vi "SequenceControl.vi"(0 "Sequence On? 2":bool, 5 "Counter 2":dbl, 7 "Sequence Instances 2":dbl, 9 "Sequence Storer":T1[][](array[typedef]) {"Amplitude Correction" step=0.1; "Line Trapping"."Phase Gradient" step=0.05; "Line Trapping"."Vector"."x" step=1e-06 format="%#_6p"; "Line Trapping"."Vector"."y" step=1e-06 format="%#_6p"; "Line Trapping"."Vector"."z" step=1e-06 format="%#_6p"; "NA Position"."r" step=1e-06; "NA Position"."y" step=1e-06; "NA Position"."x" step=1e-06; "Position"."z" step=1e-06; "Position"."y" step=1e-06; "Position"."x" step=1e-06; "Phase" step=0.7753; "Intensity" step=0.1}) -> (1 "Time per Frame (ms) 2":dbl, 2 "Sequence Order 2":dbl, 3 "Reset 2":bool, 4 "Sequence Storer 2":T1[][](array[typedef]) {"Amplitude Correction" step=0.1; "Line Trapping"."Phase Gradient" step=0.05; "Line Trapping"."Vector"."x" step=1e-06 format="%#_6p"; "Line Trapping"."Vector"."y" step=1e-06 format="%#_6p"; "Line Trapping"."Vector"."z" step=1e-06 format="%#_6p"; "NA Position"."r" step=1e-06; "NA Position"."y" step=1e-06; "NA Position"."x" step=1e-06; "Position"."z" step=1e-06; "Position"."y" step=1e-06; "Position"."x" step=1e-06; "Phase" step=0.7753; "Intensity" step=0.1}, 6 "Clearance Button 2":bool, 8 "Manual Edit 2":bool, 10 "Save State 2":bool, 12 "Play Sequence 2":bool, 13 "Bubble ID to Empty 2":dbl, 14 "Manual Sequence 2":bool, 15 "Edit Sequence Mode 2":bool)   [LabVIEW 2015]
uses:
  Matt Fall 2018 files/Matt working/Red Tweezers Image Processing Final 1-19/subvis/spot.ctl
  Matt Fall 2018 files/Matt working/Red Tweezers Image Processing Final 1-19/subvis/line_trapping.ctl
panel:
  in  "Time per Frame (ms)":dbl=500.0
  in  "Edit Sequence Mode":bool
  in  "Go to Frame":bool
  in  "Bubble ID to Empty":dbl
  in  "Clearance Button":bool
  in  "Manual Sequence":bool
  in  "Play Sequence":bool
  in  "Reset":bool
  out "Sequence Instances":dbl
  out "Counter":dbl
  in  "Save State":bool
  out "Sequence On?":bool
  in  "Sequence Order":dbl
  # "Manual Edit allows a user to\ngo to a specific sequence frame."
  # "Use this to \"clear\" a \nspecific bubble. If\nworking on a sequence,\nuse this as your delete\nbutton! You can update\nthe view by using manual edit."
  # "Use the reset button\nto clear counter.\nIt becomes necessary\nwhen you clear the array,\nespecially in manual mode."
  # "Use the sequence creator tab to specify the\nnumber of bubbles you want along with\nthe number of frames.\n\nTo save at a specific interval, the sequence\norder can be used to place the state. If used\nto correct something, it will replace the\nentire sequence frame.\n\n\"Sequence On?\" is only used in auto mode."
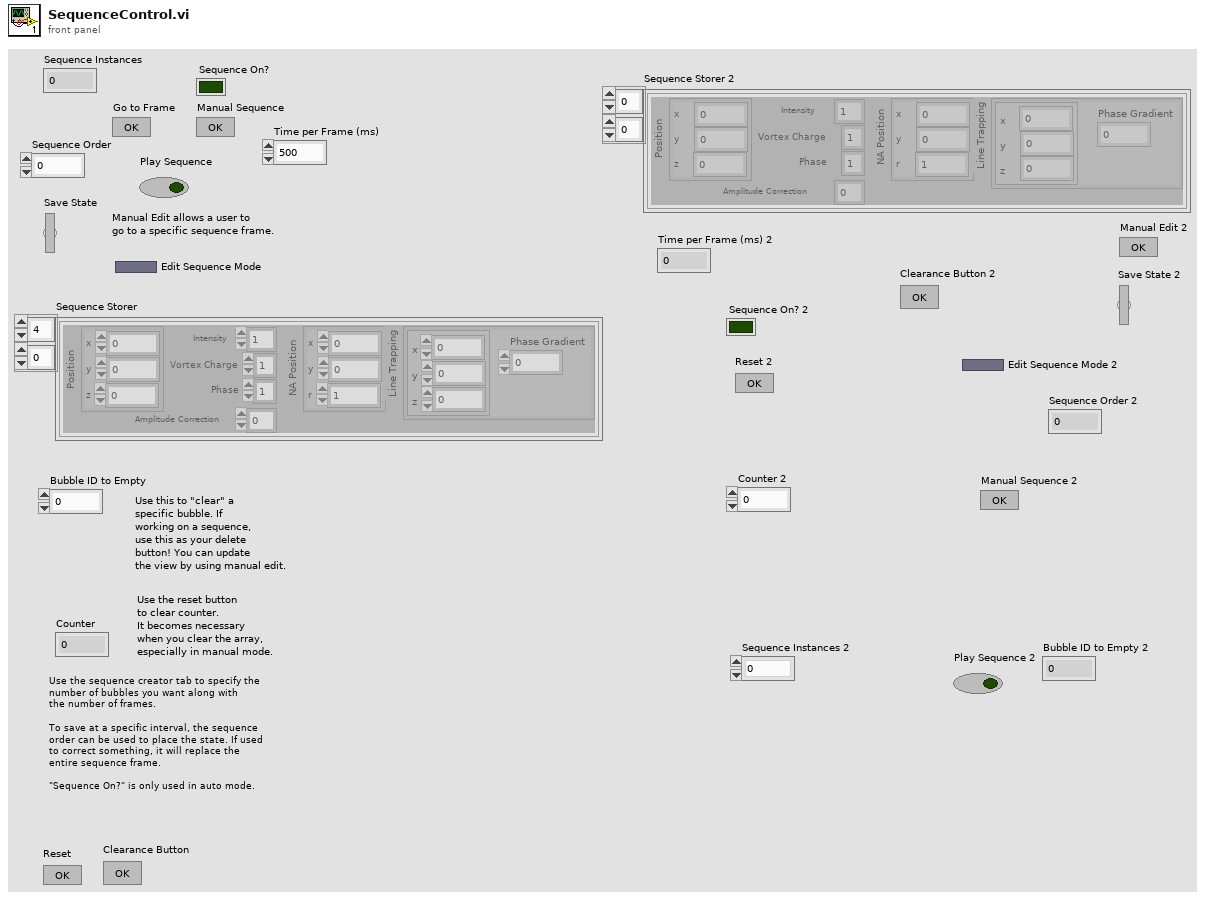
[diagram p1: front panel]
types:
  T1 = typedef "spot.ctl" = cluster{"Position":cluster{"x":dbl, "y":dbl, "z":dbl}, "Intensity":dbl, "Vortex Charge":i8, "Phase":dbl, "NA Position":cluster{"x":dbl, "y":dbl, "r":dbl}, "Line Trapping":T2, "Amplitude Correction":dbl}
  T2 = typedef "line_trapping.ctl" = cluster{"Vector":cluster{"x":dbl, "y":dbl, "z":dbl}, "Phase Gradient":dbl}
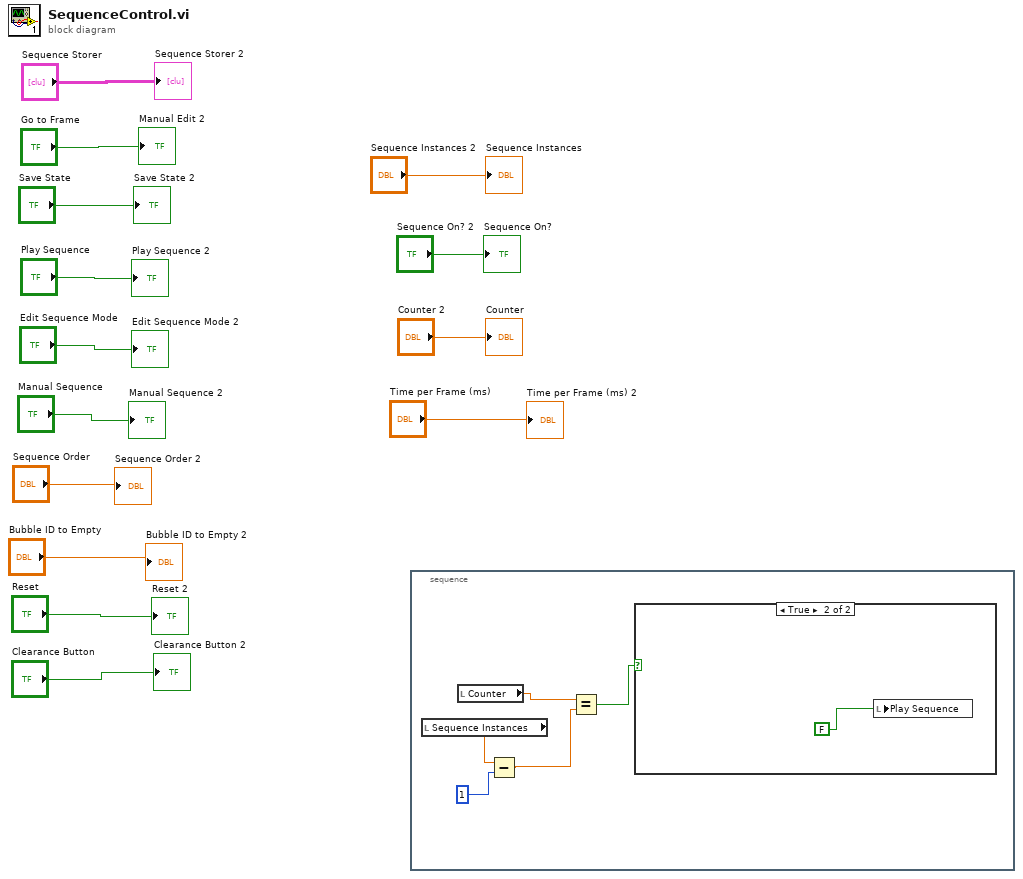
[diagram p0: block diagram]
diagram:
  n1 = stacked-sequence {
    frame #0 {
      n2 = local read "Sequence Instances"() -> (w16:dbl)
      n3 = local read "Counter"() -> (w19:dbl)
      n4 = Subtract(x=w16, y=1) -> (x-y=w17:dbl)
      n5 = Equal?(x=w19, y=w17) -> (x = y?=w18:bool)
      n6 = case shown="True" w18 {
        frame False {
        }
        frame True {
          n7 = local write "Play Sequence"(FALSE) -> ()
        }
      }
    }
  }
  "Sequence On?" <- "Sequence On? 2"
  "Counter" <- "Counter 2"
  "Sequence Instances" <- "Sequence Instances 2"
  "Sequence Storer 2" <- "Sequence Storer"
  "Manual Edit 2" <- "Go to Frame"
  "Save State 2" <- "Save State"
  "Play Sequence 2" <- "Play Sequence"
  "Edit Sequence Mode 2" <- "Edit Sequence Mode"
  "Manual Sequence 2" <- "Manual Sequence"
  "Sequence Order 2" <- "Sequence Order"
  "Bubble ID to Empty 2" <- "Bubble ID to Empty"
  "Reset 2" <- "Reset"
  "Clearance Button 2" <- "Clearance Button"
  "Time per Frame (ms) 2" <- "Time per Frame (ms)"
